vi "write_fifo_raps.vi"(8 "FIFO overflow in":bool, 9 "maximum bit depth":i8, 10 "block index in":i32, 11 "values to be written":T1) -> (0 "FIFO overflow out":bool, 2 "block index out":i32, 3 "channels out":T1)   [LabVIEW 2010]
uses:
  <vilib>/rvi/DataTransferAndStorage/Container/XNode/niFpgaContainer.xnode
  common_typedefs/channels_cluster.ctl
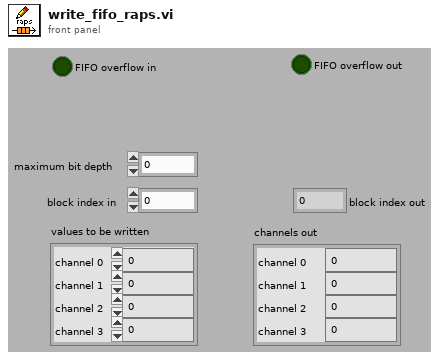
[diagram p1: front panel]
types:
  T1 = typedef "channels_cluster.ctl" = cluster{"channel 0":u32, "channel 1":u32, "channel 2":u32, "channel 3":u32}
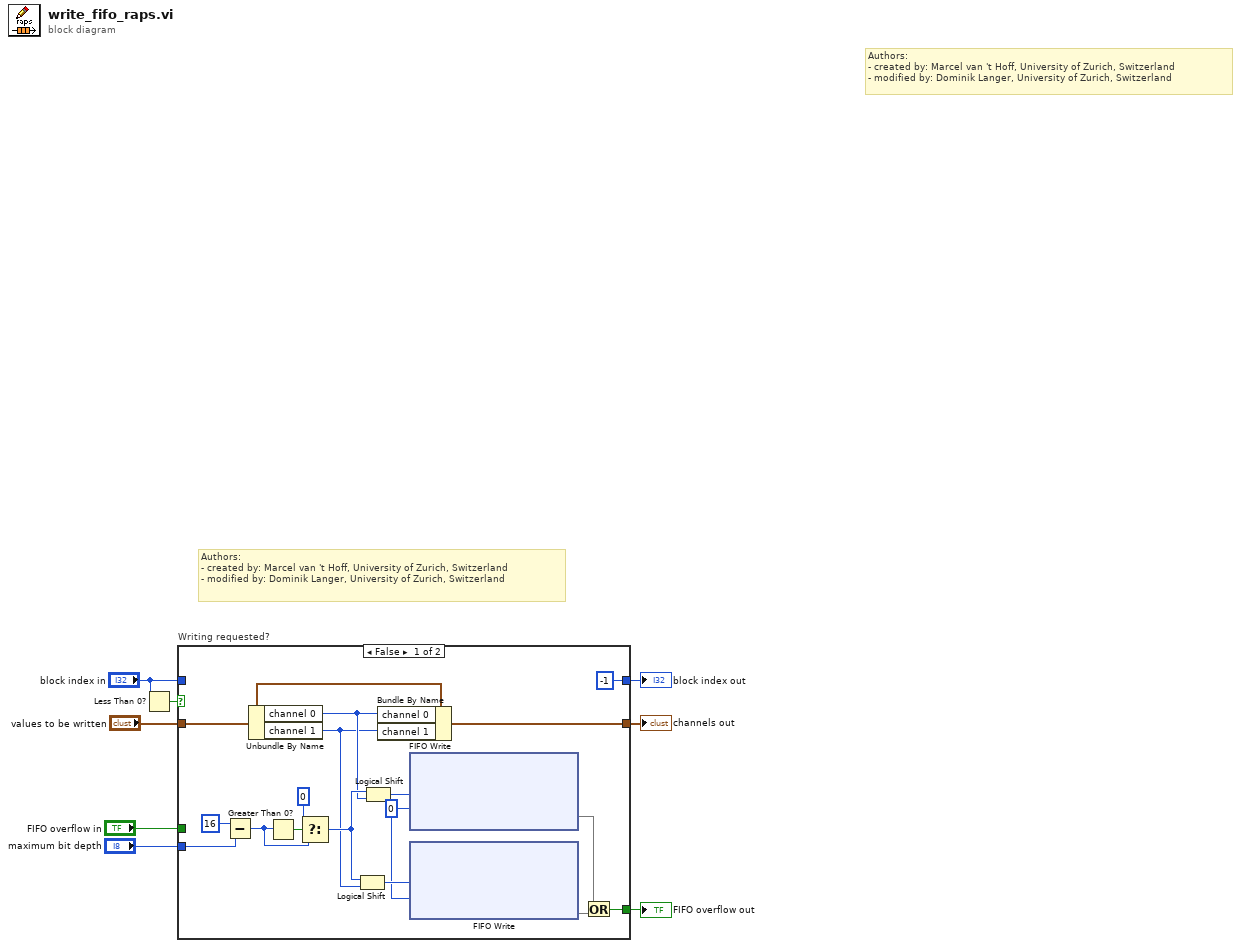
[diagram p0: block diagram]
diagram:
  # "Authors: \n- created by: Marcel van 't Hoff, University of Zurich, Switzerland\n- modified by: Dominik Langer, University of Zurich, Switzerland"
  # "Authors: \n- created by: Marcel van 't Hoff, University of Zurich, Switzerland\n- modified by: Dominik Langer, University of Zurich, Switzerland"
  n1 = Less Than 0?(x="block index in") -> (x < 0?=w4:bool)
  n2 = case "Writing requested?" shown="False" w4 {
    tunnel: [w17 w27] -> w5
    tunnel: [-1 ("block index in") w28] -> w8
    tunnel: "maximum bit depth" -> [w21 _]
    tunnel: "block index in" -> [_ w28]
    tunnel: "values to be written" -> [w16 w27]
    tunnel: "FIFO overflow in" -> [_ w26]
    tunnel: [w18 w26] -> w2
    frame False {
      w12 = 0 ("Timeout")
      n3 = Subtract(x=i8 16, y=w21) -> (x-y=w23:i8)
      n4 = Unbundle By Name(w16) -> ("channel 0"=w10:u32, "channel 1"=w9:u32)
      n5 = Greater Than 0?(x=w23) -> (x > 0?=w22:bool)
      n6 = Select(t=i8 0 ("f"), s=w22, f=w23) -> (s? t:f=w13:i8)
      n7 = Logical Shift(y=w13, x=w9) -> (x << y=w15:u32)
      n8 = Logical Shift(y=w13, x=w10) -> (x << y=w14:u32)
      n9 = Bundle By Name(cluster=w16, "channel 0"=w10, "channel 1"=w9) -> (w17:T1)
      n10 = xnode ("FIFO Write")("Element"=w14, "Timeout"=w12) -> ("Timed Out?"=w19)  [unwired: 1 in, 1 out]
      n11 = xnode ("FIFO Write")("Element"=w15, "Timeout"=w12) -> ("Timed Out?"=w20)  [unwired: 1 in, 1 out]
      n12 = Or(x=w19, y=w20) -> (x .or. y?=w18:bool)
    }
    frame True {
    }
  }
  "channels out" <- w5
  "block index out" <- w8
  "FIFO overflow out" <- w2
